vi "XBee_Continuous.vi"(0 "VISA resource name":refnum<visa-resource-name>="COM1", 1 "baud rate":u32=9600, 4 "data bits":u16=8 min=5 max=8 step=1, 5 "parity":u16(ring) items=["None", "Odd", "Even", "Mark", "Space"], 7 "stop bits":u16=10, 9 "XON Character":u8=17 format="%.0x", 14 "XOFF Character":u8=19 format="%.0x", 15 "timeout (ms)":u32=10000, 21 "End read on termination character?":bool, 24 "termination char\n(0xA = '\\n' = LF)":u8=10 format="%.0x", 25 "buffer size":u32=4096) -> ()   [LabVIEW 2015]
doc: "The Advanced Serial Read and Write example performs a Serial Port Read, a Serial Port Write, or a combination of these actions while setting some advanced serial features like buffer size, termination characters, and XON/XOFF flow control. The user selects the actions (read or write) on the front panel. If both are selected, the VI will write the data first, read the data and then close the VISA session that is opened to the port. \n\nThe parameters set for the serial port must match the parameters of the connected instrument or device. In this example, the bytes to read parameter specifies the number of bytes that the serial port reads. If there were more bytes at the port than the number specified in bytes to read, those bytes would not be read. Also, if you specify to read more bytes than the number of bytes actually read, you might receive a timeout error message.\n\nINSTRUCTIONS:\n1) Select the serial resource and configuration parameters (baud rate, data bits, parity, stop bits, flow control).\n2) Termination character can be enabled and set. Also, set the required input buffer size prior to running the example.\n3) Select the operations to be performed. \n4) Connect the serial port to your device. If no device is available, perform a loopback test by doing one of the following. Short pins 2 and 3 on a RS-232 cable or short pin 4 to pin 8 and pin 5 to pin 9 on a RS-485/422 cable. \n5) Run the VI to see the data read. (The \"read string\" will match the \"string to write\" if a loopback test was performed.)\n\nThis example exposes several advanced features that you may need for your application. Not all applications need all the features shown in this example. The input buffer size is likely an important setting that you want to control in your application. This example expands upon the flow control option for XON and XOFF, allowing the user to choose those control characters. The timeout parameter has been brought to the front panel so a user can specify the time period the VISA Read will wait for the number of bytes to read before timing out. Also, the user has several controls for the termination character, which is discussed later.\n\nNote that you can press the write and read buttons and change the bytes to read parameters on the fly, while the example is running. However, you must stop the example to change the other configuration parameters after the example has started running, and then run again.\n\nSet the I/O buffer size slightly higher the amount of data you expect to receive. This is very important for applications that don't use flow control, as you may lose characters if the receive buffer overflows.\n\nSetting the timeout period ensures that the operation returns with a timeout error if the operation cannot be performed in the specified time period. \n\nSome devices require a termination character in order to identify the end of command strings. Some devices send a termination character to signify the end of data to be read. \n\nThis example shows how you can end the Read operation once a termination character is detected in the buffer and/or append a termination character at the end of the Write data. To enable the Read to end on a termination character, use the VISA Configure Serial Port or use the VISA Properties Serial End Mode for Reads, Termination Character Enable, and Termination Character. To end the Write with a termination character, use the VISA Properties Serial End Mode for Writes, the Send End Enable, and Termination Character. In this example, the same termination character is used for both the Read and the Write. You can specify two different characters for your application, if desired.\n\nYour application may require specific characters for the XON/XOFF Flow Control. You can specify these characters with the VISA Properties Flow Control XOFF Character and Flow Control XON Character. Note that if the standard XON and XOFF characters are used, then decimal 17 and 19 are unavailable for data values. Remember that using flow control and setting an adequate buffer size allow you to prevent buffer overflows."
uses:
  <vilib>/Analysis/2dsp.llb/Complex FFT.vi
  <vilib>/Instr/_visa.llb/VISA Configure Serial Port (Instr).vi
  <vilib>/measure/madcrms.llb/Basic Averaged DC-RMS for 1 Chan.vi
  <vilib>/measure/NI_MAPro.lvlib
  <vilib>/Analysis/NI_AALPro.lvlib
panel:
  in  "time":timestamp=timestamp(3198752888.296 s since 1904-01-01)
  out "I/Q channels":dynamicdata(graph)
  out "Spectrum":waveform(dbl)(graph)
  in  "Save raw data":bool
  in  "Data saving path":path=path "C:/Users/zpeng/OneDrive - Texas Tech University/Desktop"
  in  "radar ID":u8=1
  in  "FFT":i32=1024
  in  "flow control":u16(ring) items=["None"=0, "XON/XOFF"=1, "RTS/CTS"=2, "DTR/DSR"=4]
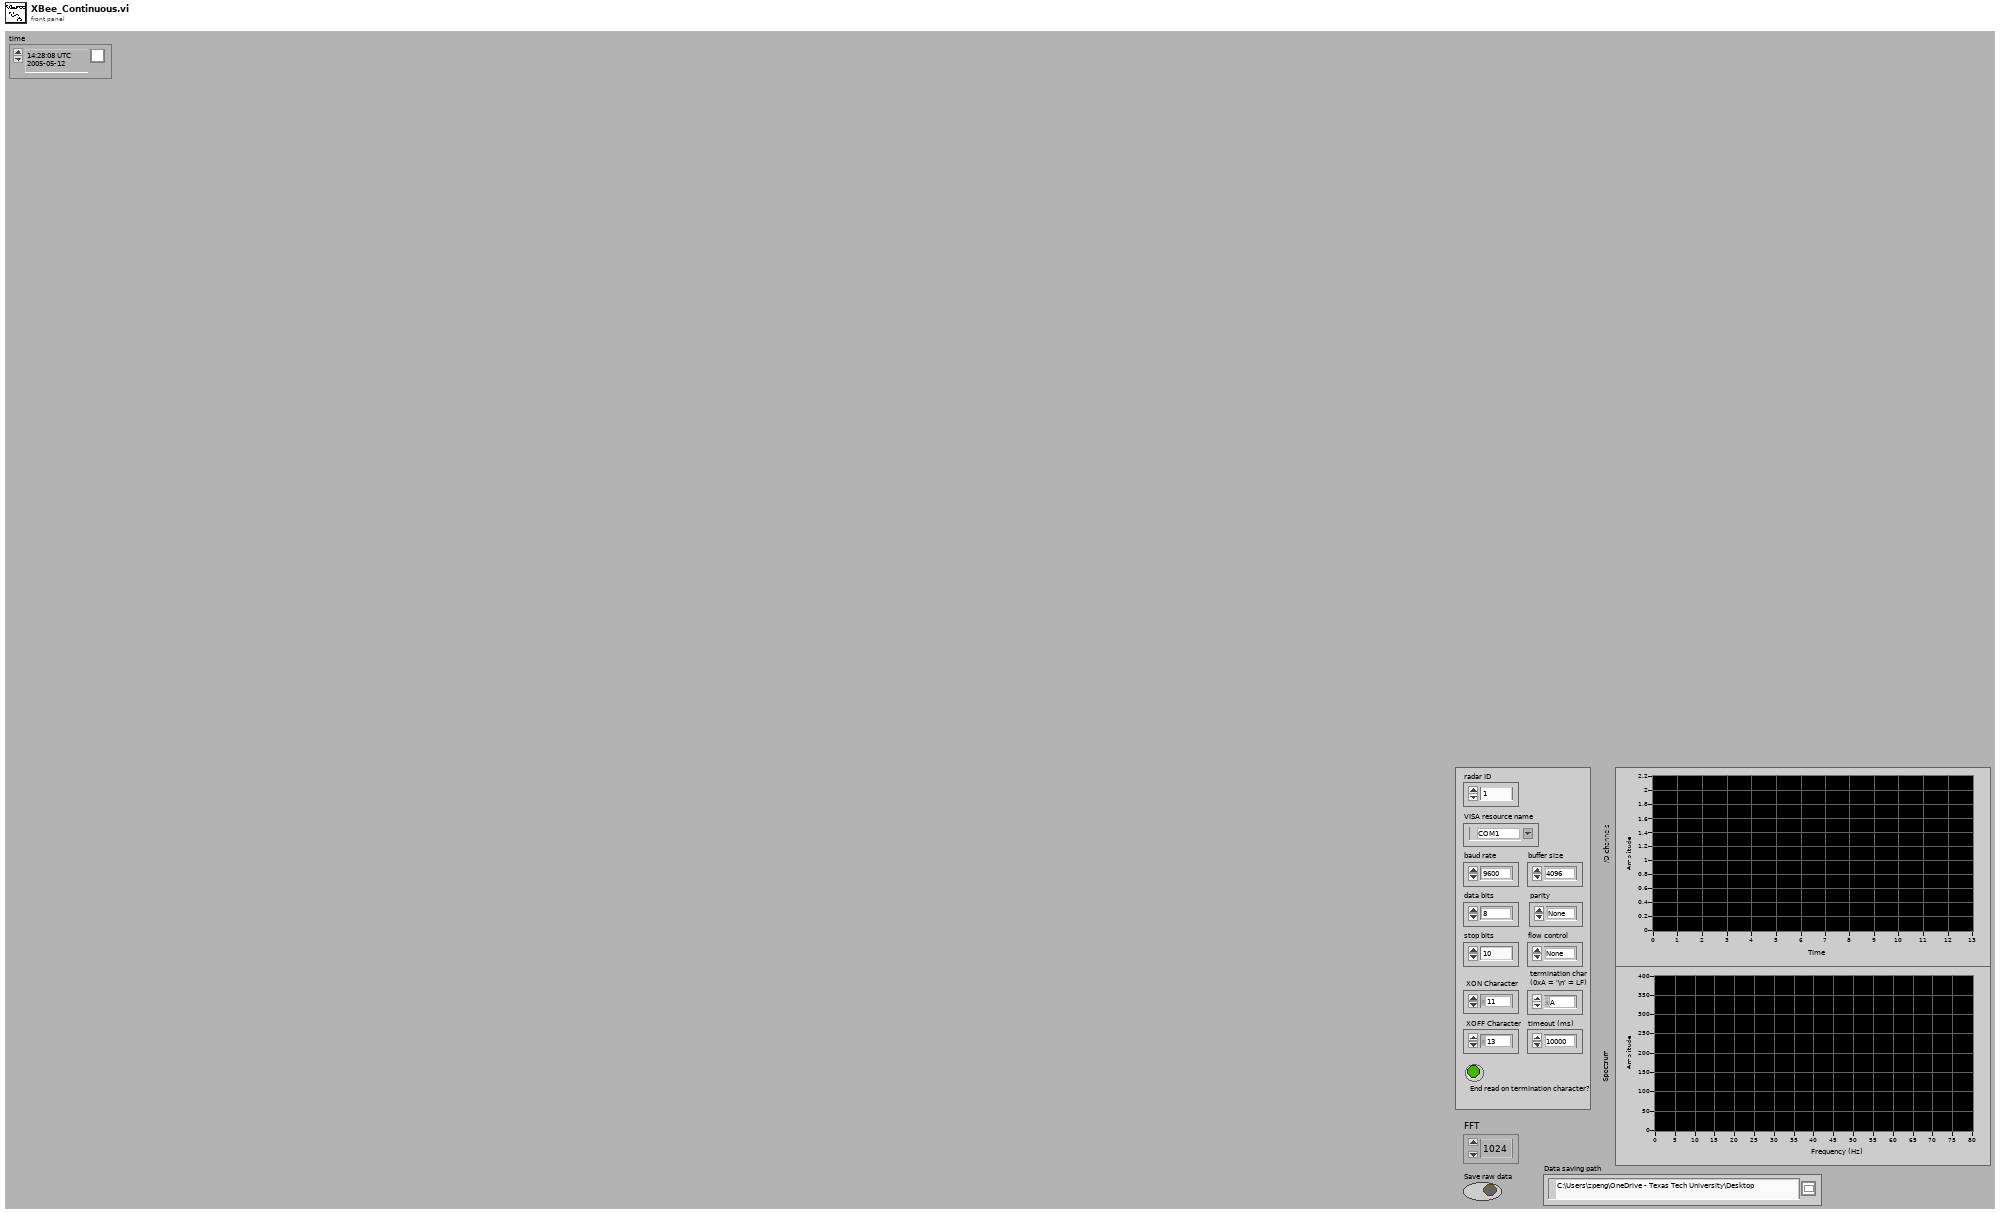
[diagram p1: front panel]
types:
  T1 = enum16{"open", "replace", "create", "open or create", "replace or create", "replace or create with confirmation"}
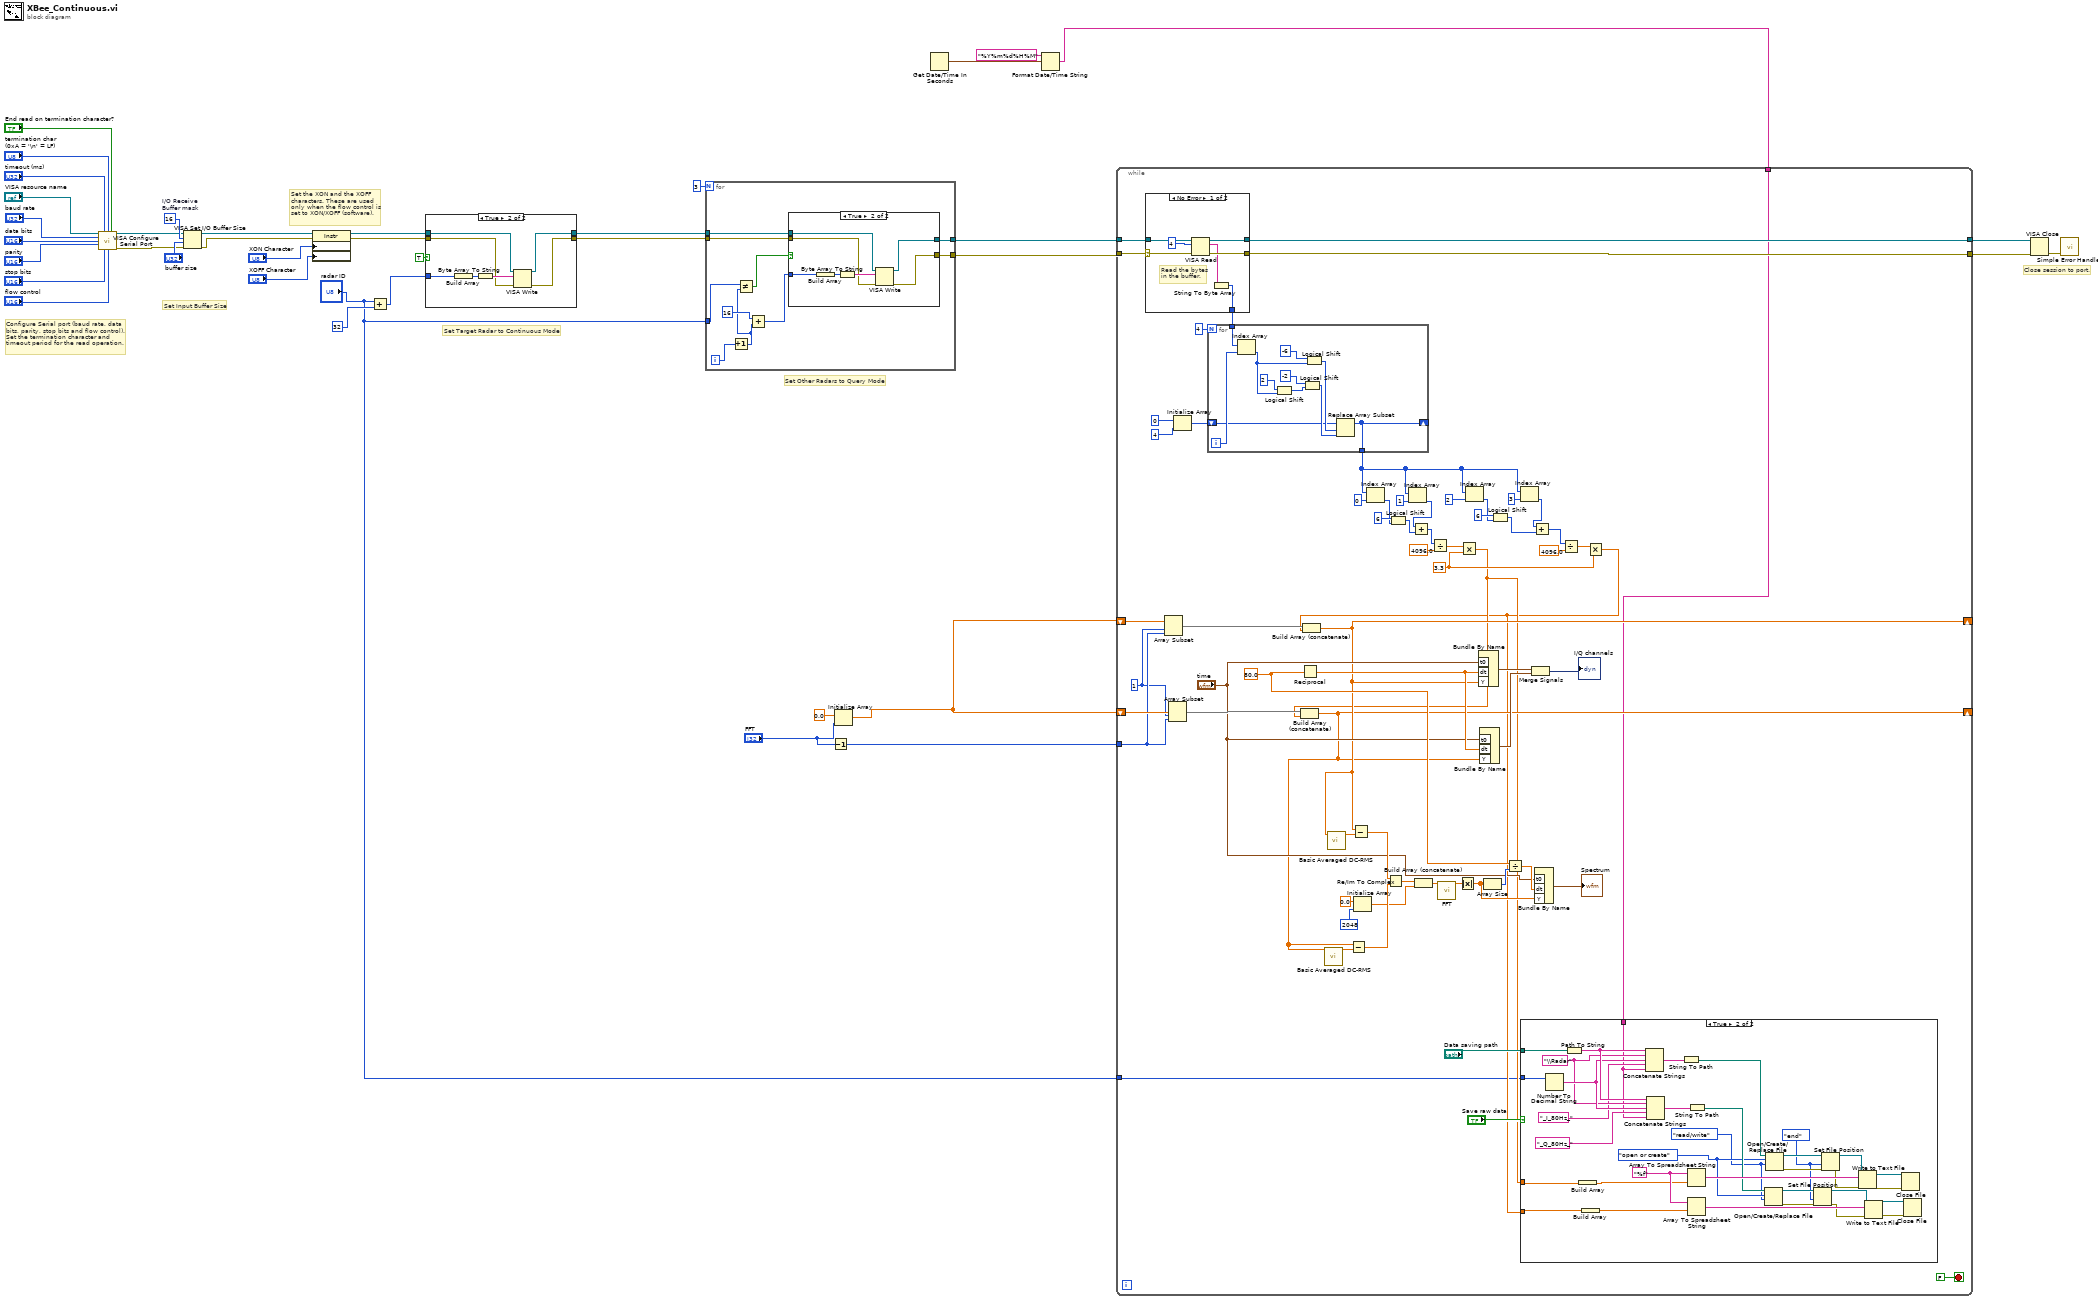
[diagram p0: block diagram]
diagram:
  w31 = u16 16  # I/O Receive Buffer mask
  # "Set Other Radars to Query Mode"
  # "Set Target Radar to Continuous Mode"
  # "Set the XON and the XOFF\ncharacters. These are used\nonly when the flow control is\nset to XON/XOFF (software)."
  # "Configure Serial port (baud rate, data\nbits, parity, stop bits and flow control).\nSet the termination character and\ntimeout period for the read operation."
  # "Set Input Buffer Size"
  # "Close session to port."
  n1 = call-poly "VISA Configure Serial Port"("VISA resource name"="VISA resource name", "timeout (10sec)"="timeout (ms)", "termination char\n(0xA = '\\n' = LF)"="termination char\n(0xA = '\\n' = LF)", "Enable Termination\nChar (T)"="End read on termination character?", "baud rate (9600)"="baud rate", "data bits (8)"="data bits", "parity (0:none)"="parity", "stop bits (10: 1 bit)"="stop bits", "flow control (0:none)"="flow control") -> ("VISA resource name out"=w20:refnum<visa-resource-name>, "error out"=w19:errorcluster)  [unwired: 1 in, 4 out]
  n2 = VISA Set I/O Buffer Size(VISA resource name=w20, mask (16)=w31, size (4096)="buffer size", error in (no error)=w19) -> (VISA resource name out=w27:refnum<visa-resource-name>, error out=w26:errorcluster)
  n3 = property class="Instr"(reference=w27, error in=w26, "Serial Settings:Flow Control XON Character"="XON Character", "Serial Settings:Flow Control XOFF Character"="XOFF Character") -> (reference out=w16:refnum<visa-resource-name>, error out=w15:errorcluster)
  n4 = Add(x="radar ID", y=u8 32 ("element")) -> (x+y=w12:u8)
  n5 = case shown="True" TRUE {
    tunnel: w15 -> [w40 w46]
    tunnel: w16 -> [w39 w45]
    tunnel: [w39 w44] -> w10
    tunnel: [w40 w43] -> w9
    tunnel: w12 -> [_ w41]
    frame False {
    }
    frame True {
      n6 = Build Array(w41) -> (w42:u8[])
      n7 = Byte Array To String(unsigned byte array=w42) -> (string=w47:string)
      n8 = VISA Write(VISA resource name=w45, write buffer=w47, error in (no error)=w46) -> (VISA resource name out=w44:refnum<visa-resource-name>, error out=w43:errorcluster)  [unwired: 1 out]
    }
  }
  n9 = for {
    N: 3 -> [_]
    tunnel: w10 -> [w54]
    tunnel: w9 -> [w48]
    tunnel: "radar ID" -> [w53]
    tunnel: [w50] -> w8
    tunnel: [w49] -> w7
    i -> [w56]
    n10 = Increment(x=w56) -> (x+1=w52:i32)
    n11 = Not Equal?(x=w53, y=w52) -> (x != y?=w51:bool)
    n12 = Add(x=u8 16 ("element"), y=w52) -> (x+y=w55:i32)
    n13 = case shown="True" w51 {
      tunnel: w48 -> [w59 w65]
      tunnel: w54 -> [w58 w64]
      tunnel: [w58 w63] -> w50
      tunnel: [w59 w62] -> w49
      tunnel: w55 -> [_ w60]
      frame False {
      }
      frame True {
        n14 = Build Array(w60) -> (w61:i32[])
        n15 = Byte Array To String(unsigned byte array=w61) -> (string=w66:string)
        n16 = VISA Write(VISA resource name=w64, write buffer=w66, error in (no error)=w65) -> (VISA resource name out=w63:refnum<visa-resource-name>, error out=w62:errorcluster)  [unwired: 1 out]
      }
    }
  }
  n17 = Decrement(x="FFT") -> (x-1=w5:i32)
  n18 = Initialize Array(0.0 ("element"), "FFT") -> (w6:dbl[])
  n19 = Get Date/Time In Seconds() -> (seconds since 1Jan1904=w17:timestamp)
  n20 = Format Date/Time String(time format string (%c)="%Y%m%d%H%M", seconds (now)=w17) -> (date/time string=w4:string)  [unwired: 1 in]
  n21 = while {
    tunnel: w7 -> [w102]
    tunnel: w8 -> [w101]
    tunnel: [w76] -> w3
    tunnel: [w75] -> w2
    tunnel: w5 -> [w114]
    shift-right: [w81] -> _
    shift-left: w6 -> [w129]
    shift-right: [w82] -> _
    shift-left: w6 -> [w115]
    tunnel: w4 -> [w71]
    tunnel: "radar ID" -> [w67]
    stop <- FALSE stop-if-true
    w83 = 1 ("index")
    (unwired) 0
    w107 = 3.3 ("y")
    w91 = 80.0 ("dt")
    n22 = case "Read bytes from port." shown="No Error" w102 {
      selector: w102 -> [w179 w184]
      tunnel: [w181 w184] -> w75
      tunnel: [w182 w185] -> w76
      tunnel: w101 -> [w180 w185]
      tunnel: [w177 u8[] [] ("unsigned byte array")] -> w77
      frame No Error {
        # "Read the bytes\nin the buffer."
        n23 = VISA Read(VISA resource name=w180, byte count=u32 4, error in (no error)=w179) -> (VISA resource name out=w182:refnum<visa-resource-name>, read buffer=w178:string, error out=w181:errorcluster)  [unwired: 1 out]
        n24 = String To Byte Array(string=w178) -> (unsigned byte array=w177:u8[])
      }
      frame Error {
        # "Error occurred \nreading Bytes at \nSerial Port"
      }
    }
    n25 = Array Subset(array=w115, index=w83, length=w114) -> (w116:dbl[])
    n26 = Array Subset(array=w129, index=w83, length=w114) -> (w130:dbl[])
    n27 = Initialize Array(i16 0 ("element"), 4 ("dimension size")) -> (w78:i16[])
    n28 = for {
      N: 4 -> [_]
      tunnel: w77 -> [w170]
      tunnel: [w165] -> w84
      shift-right: [w165] -> _
      shift-left: w78 -> [w166]
      i -> [w169]
      n29 = Index Array(array=w170, index=w169) -> (element=w173:u8)
      n30 = Logical Shift(y=i8 2, x=w173) -> (x << y=w172:u8)
      n31 = Logical Shift(y=i8 -2, x=w172) -> (x << y=w167:u8)
      n32 = Logical Shift(y=i8 -6, x=w173) -> (x << y=w168:u8)
      n33 = Replace Array Subset(array=w166, new element=w167, index=w168) -> (w165:i16[])
    }
    n34 = Reciprocal(x=w91) -> (1/x=w105:dbl)
    n35 = Initialize Array(0.0 ("element"), 2048 ("dimension size")) -> (w95:dbl[])
    n36 = Index Array(array=w84, index=0) -> (element=w123:i16)
    n37 = Logical Shift(y=i16 6, x=w123) -> (x << y=w119:i16)
    n38 = Index Array(array=w84, index=1) -> (element=w120:i16)
    n39 = Add(x=w120, y=w119) -> (x+y=w74:i16)
    n40 = Divide(x=w74, y=4096.0) -> (x/y=w112:dbl)
    n41 = Multiply(x=w112, y=w107) -> (x*y=w70:dbl)
    n42 = Build Array (concatenate)(w130, w70) -> (w81:dbl[])
    n43 = call-poly <vilib>:"Basic Averaged DC-RMS.vi"("signal in"=w81) -> ("DC value"=w108:dbl)  [unwired: 4 in, 6 out]
    n44 = Subtract(x=w81, y=w108) -> (x-y=w99:dbl[])
    n45 = Index Array(array=w84, index=2) -> (element=w121:i16)
    n46 = Bundle By Name ("Build Waveform")("t0"="time", "dt"=w105, "Y"=w81) -> (w103:waveform(dbl))  [unwired: 1 out]
    n47 = Logical Shift(y=i16 6, x=w121) -> (x << y=w117:i16)
    n48 = Index Array(array=w84, index=3) -> (element=w118:i16)
    n49 = Add(x=w118, y=w117) -> (x+y=w86:i16)
    n50 = Divide(x=w86, y=4096.0) -> (x/y=w110:dbl)
    n51 = Multiply(x=w110, y=w107) -> (x*y=w69:dbl)
    n52 = Build Array (concatenate)(w116, w69) -> (w82:dbl[])
    n53 = call-poly <vilib>:"Basic Averaged DC-RMS.vi"("signal in"=w82) -> ("DC value"=w109:dbl)  [unwired: 4 in, 6 out]
    n54 = Subtract(x=w82, y=w109) -> (x-y=w100:dbl[])
    n55 = Re/Im To Complex(1:w99, 2:w100) -> (0:w94:cdb[])
    n56 = Build Array (concatenate)(w94, w95) -> (w96:cdb[])
    n57 = call-poly <vilib>:"FFT.vi"("X"=w96) -> ("FFT {X}"=w92:cdb[])  [unwired: 2 in, 8 out]
    n58 = Absolute Value(x=w92) -> (abs(x)=w90:dbl[])
    n59 = Bundle By Name ("Build Waveform")("t0"="time", "dt"=w105, "Y"=w82) -> (w104:waveform(dbl))  [unwired: 1 out]
    n60 = Array Size(array=w90) -> (size(s)=w93:i32)
    n61 = Divide(x=w91, y=w93) -> (x/y=w89:dbl)
    n62 = case shown="True" "Save raw data" {
      tunnel: w70 -> [_ w157]
      tunnel: w69 -> [_ w138]
      tunnel: w71 -> [_ w131]
      tunnel: "Data saving path" -> [_ w158]
      tunnel: w67 -> [_ w136]
      frame False {
      }
      frame True {
        w139 = enum16{"read/write", "read-only", "write-only"}."read/write" ("access (0:read/write)")
        w140 = T1."open or create" ("operation (0:open)")
        w148 = enum16{"start", "end", "current"}."end" ("from (0:start)")
        w134 = "\\Radar" ("string")
        w160 = "%f" ("format string")
        n63 = Number To Decimal String(number=w136) -> (decimal integer string=w135:string)  [unwired: 1 in]
        n64 = Path To String(path=w158) -> (string=w162:string)
        n65 = Build Array(w157) -> (w137:dbl[])
        n66 = Build Array(w138) -> (w156:dbl[])
        n67 = Concatenate Strings(w162, w134, w135, "_I_80Hz_" ("string"), w131) -> (w164:string)
        n68 = Concatenate Strings(w162, w134, w135, "_Q_80Hz_" ("string"), w131) -> (w161:string)
        n69 = String To Path(string=w164) -> (path=w155:path)
        n70 = Array To Spreadsheet String(array=w137, 3:w160) -> (spreadsheet string=w163:string)  [unwired: 1 in]
        n71 = Array To Spreadsheet String(array=w156, 3:w160) -> (spreadsheet string=w159:string)  [unwired: 1 in]
        n72 = String To Path(string=w161) -> (path=w154:path)
        n73 = Open/Create/Replace File(file path (use dialog)=w154, operation (0:open)=w140, access (0:read/write)=w139) -> (refnum out=w149:refnum<file>, error out=w147:errorcluster)  [unwired: 3 in, 1 out]
        n74 = Open/Create/Replace File(file path (use dialog)=w155, operation (0:open)=w140, access (0:read/write)=w139) -> (refnum out=w153:refnum<file>, error out=w152:errorcluster)  [unwired: 3 in, 1 out]
        n75 = Set File Position(refnum=w149, from (0:start)=w148, error in=w147) -> (refnum out=w145:refnum<file>, error out=w146:errorcluster)  [unwired: 1 in]
        n76 = Set File Position(refnum=w153, from (0:start)=w148, error in=w152) -> (refnum out=w151:refnum<file>, error out=w150:errorcluster)  [unwired: 1 in]
        n77 = Write to Text File(file (use dialog)=w151, text=w163, error in=w150) -> (refnum out=w144:refnum<file>, error out=w143:errorcluster)  [unwired: 1 in, 1 out]
        n78 = Write to Text File(file (use dialog)=w145, text=w159, error in=w146) -> (refnum out=w142:refnum<file>, error out=w141:errorcluster)  [unwired: 1 in, 1 out]
        n79 = Close File(refnum=w144, error in=w143) -> ()  [unwired: 2 out]
        n80 = Close File(refnum=w142, error in=w141) -> ()  [unwired: 2 out]
      }
    }
    n81 = Merge Signals(w104, w103) -> (→"I/Q channels":dynamicdata)
    n82 = Bundle By Name("t0"="time", "dt"=w89, "Y"=w90) -> (→"Spectrum":waveform(dbl))  [unwired: 1 out]
  }
  n83 = VISA Close(VISA resource name=w3, error in (no error)=w2) -> (error out=w36:errorcluster)
  n84 = call <vilib>:"Simple Error Handler.vi"("error in (no error)"=w36) -> ()  [unwired: 1 in, 8 out]
